vi "Cache-BroadcastReg(NonCSM).vi"(8 "error in (no error)":errorcluster, 10 "CSM Name":string, 11 "Broadcast State":string) -> (0 "error out":errorcluster, 3 "Array":T2(array[cluster]))   [LabVIEW 2017, in "Communicable State Machine.lvlib"]
doc: "### Cache-Broadcast Registry Search Result.vi\n\n-- <b>Controls</b> --\n- <b>CSM Name</b>:\n- <b>Broadcast state</b>:\n\n-- <b>Indicators</b> --\n- <b>Array</b>:"
uses:
  Communicable State Machine.lvlib
  AdvanceAPI/CSM - Broadcast Message Type.ctl
  Operation-BroadcastRegistry.ctl
  ChangeFlag/ChangeFlag-Read.vi
  ChangeFlag/ChangeFlagDB.vi
  _Shared/CSM Shared.lvlib
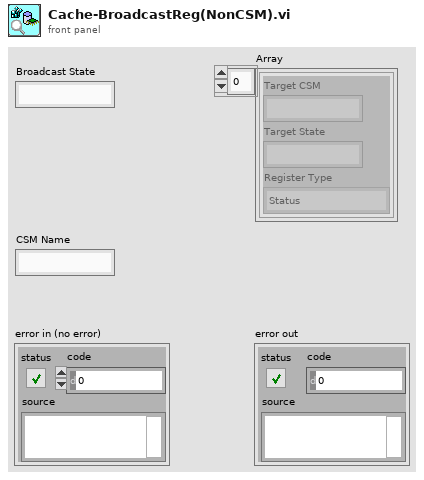
[diagram p1: front panel]
types:
  T1 = typedef "Communicable State Machine.lvlib/CSM - Broadcast Message Type.ctl" = enum16{"<Null>", "Status", "Interrupt"}
  T2 = cluster{"Target CSM":string, "Target State":string, "Register Type":T1}[]
  T3 = cluster{"Target CSM":string, "Target State":string, "Register Type":T1}
  T4 = typedef "Communicable State Machine.lvlib/Operation-BroadcastRegistry.ctl" = enum16{"Delete Source Module", "Delete Target Module", "Remove Module", "Register", "Unregister", "Check", "List Status", "List Entries", "List Status Of Source", "Drop", "Register As Status", "Register As Interrupt"}
  T5 = typedef "Communicable State Machine.lvlib/BroadcastRegistry-Value.ctl" = cluster{"Name":string, "Register Type":T1}
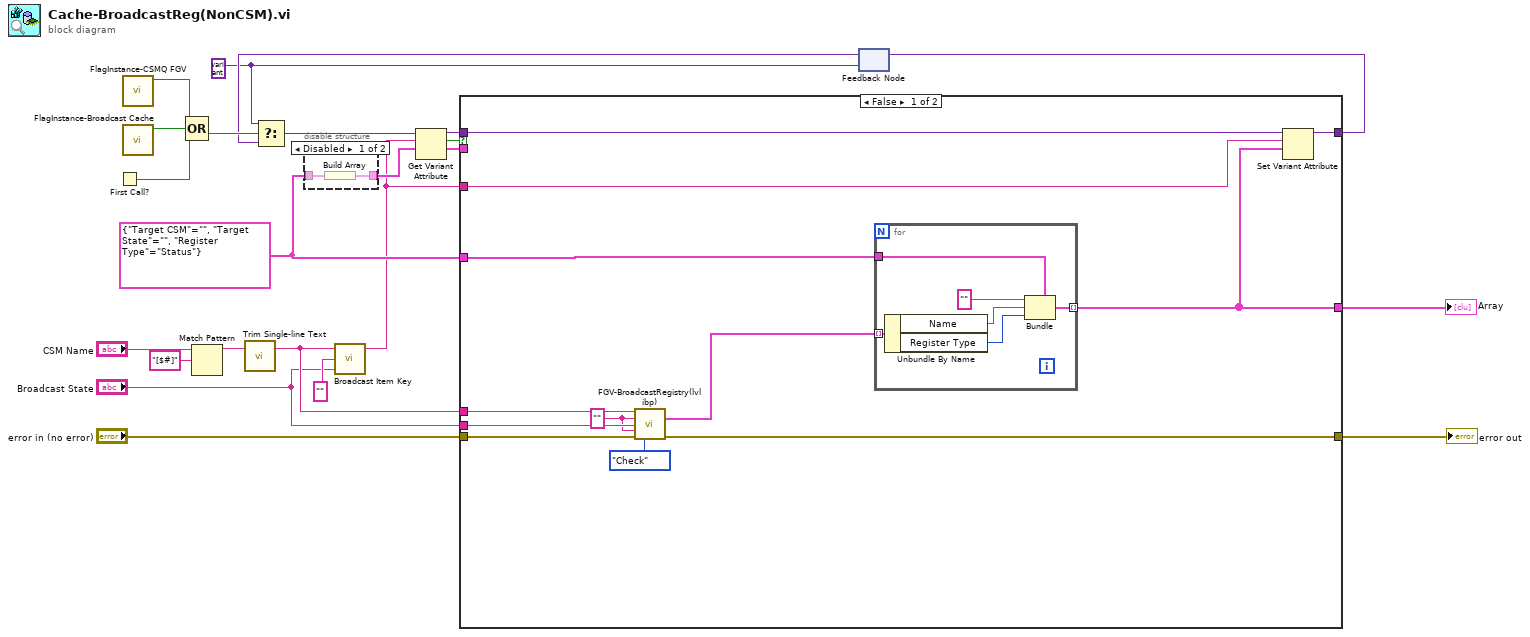
[diagram p0: block diagram]
diagram:
  w15 = T3 {"Target CSM"="", "Target State"="", "Register Type"=enum."Status"} ("cluster")
  w17 = variant
  n1 = First Call?() -> (First Call?: T/F=w20:bool)
  n2 = call "FlagInstance-CSMQ FGV.vi"() -> ("Changed"=w2:bool)  [unwired: 10 in, 1 out]
  n3 = call "FlagInstance-Broadcast Cache.vi"() -> ("Changed"=w1:bool)  [unwired: 10 in, 1 out]
  n4 = Compound Arithmetic op=OR(w2, w1, w20) -> (w19:bool)
  n5 = Match Pattern(string="CSM Name", regular expression="[$#]") -> (before substring=w8:string)  [unwired: 1 in, 3 out]
  n6 = call "Trim Single-line Text.vi"("single-line text"=w8) -> ("trimed text"=w6:string)  [unwired: 2 in]
  n7 = disable-structure shown="Disabled" {
    disable-tunnel: w15 -> [w25 _]
    disable-tunnel: [w24 _] -> w14
    frame Disabled {
      n8 = Build Array(w25) -> (w24:T2)
    }
    frame Enabled {
    }
  }
  n9 = call "Broadcast Item Key.vi"("Status"="Broadcast State", "Target"="" ("target"), "Source"=w6) -> ("Key"=w3:string)  [unwired: 2 in]
  n10 = feedback #1(w17) -> (w18:variant)
  n11 = Select(t=w17, s=w19, f=w18) -> (s? t:f=w16:variant)
  n12 = Get Variant Attribute(Variant=w16, name=w3, default value (empty Variant)=w14) -> (duplicate Variant=w12:variant, found=w13:bool, value=w11:T2)  [unwired: 1 in, 1 out]
  n13 = case shown="False" w13 {
    tunnel: [w37 w45] -> w23
    tunnel: "error in (no error)" -> [w29 w45]
    tunnel: [w31 w46] -> w21
    tunnel: "Broadcast State" -> [w36 _]
    tunnel: w6 -> [w35 _]
    tunnel: w15 -> [w34 _]
    tunnel: w12 -> [w33 w44]
    tunnel: w11 -> [_ w46]
    tunnel: w3 -> [w32 _]
    tunnel: [w30 w44] -> w10
    frame False {
      w26 = "" ("Target")
      n14 = call "FGV-BroadcastRegistry(lvlibp).vi"("Source"=w35, "Target"=w26, "Status"=w36, "API"=w26, "Error In"=w29, "Operation"=Operation-BroadcastRegistry."Check") -> ("Values"=w27:T5[], "error out"=w37:errorcluster)  [unwired: 7 in, 1 out]
      n15 = for {
        tunnel: w34 -> [w42]
        tunnel: [w43] -> w31 mode=indexing
        tunnel: w27 -> [w41] mode=indexing
        n16 = Unbundle By Name(w41) -> ("Name"=w40:string, "Register Type"=w39:T1)
        n17 = Bundle(cluster=w42, "Target CSM"="", "Target State"=w40, "Register Type"=w39) -> (w43:T3)
      }
      n18 = Set Variant Attribute(Variant=w33, name=w32, value=w31) -> (Variant out=w30:variant)  [unwired: 1 in, 2 out]
    }
    frame True {
    }
  }
  "error out" <- w23
  "Array" <- w21
  n19 = feedback-in #1(w10) -> ()
